vi "SearchArrayPath.vi"(6 "Current Direction (T=Positive)":bool=TRUE, 7 "Current Pos":T2, 8 "Target":T3, 9 "Blacklist":cluster{"X":dbl, "Y":dbl, "Z":dbl}[](array[cluster]), 10 "Path Taken":T1[](array[typedef]), 11 "All Lines":T4) -> (1 "Found Path?":bool, 2 "Path taken":T1[][](array[typedef]))   [LabVIEW 2014, in "Map Data.lvlib"]
uses:
  Map Data.lvlib
  All-Lines.ctl
  LineCluster.ctl
  LineConnection.ctl
  Components/PathFinder/Controls/PathControl.ctl
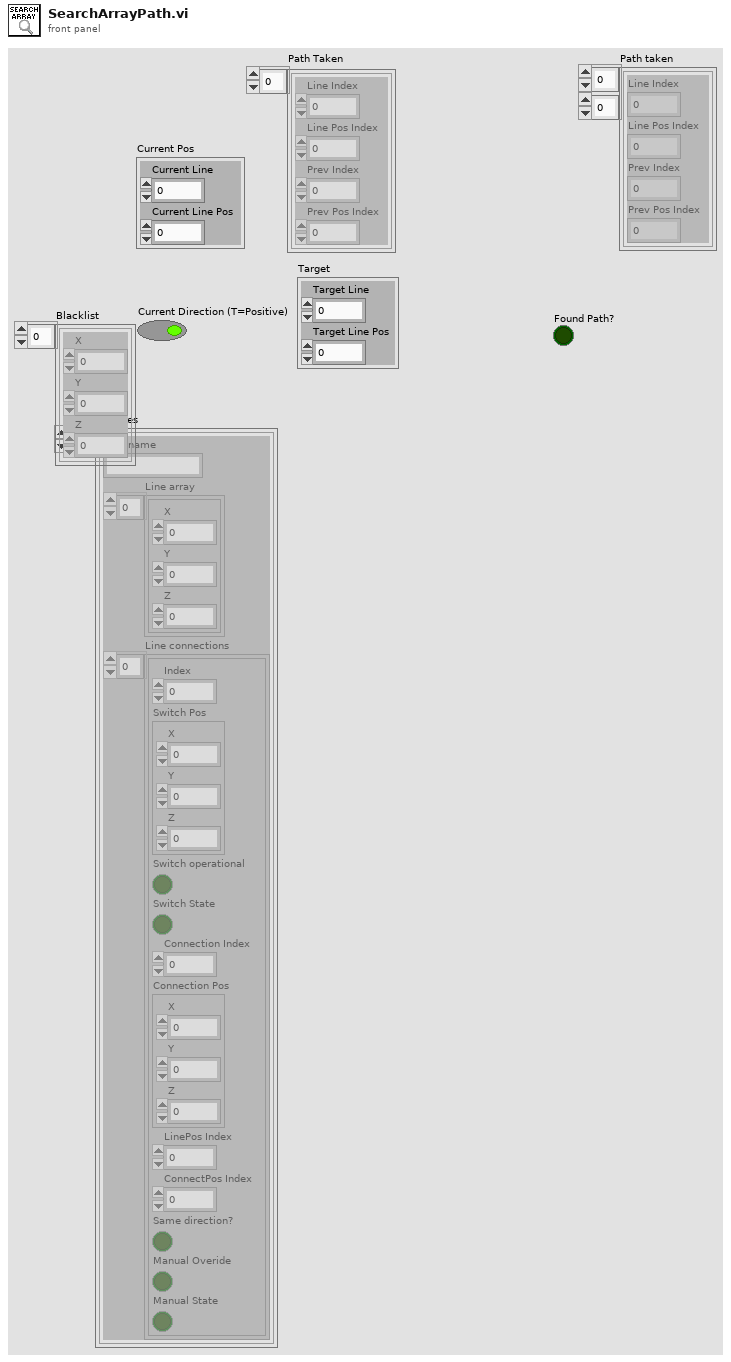
[diagram p1: front panel]
types:
  T1 = typedef "PathControl.ctl" = cluster{"Line Index":i32, "Line Pos Index ":i32, "Prev Index ":i32, "Prev Pos Index":i32}
  T2 = cluster{"Current Line":i32, "Current Line Pos":i32}
  T3 = cluster{"Target Line":i32, "Target Line Pos":i32}
  T4 = typedef "Map Data.lvlib/All-Lines.ctl" = T5[]
  T5 = typedef "Map Data.lvlib/LineCluster.ctl" = cluster{"Line name":string, "Line array":cluster{"X":dbl, "Y":dbl, "Z":dbl}[], "Line connections":T6[]}
  T6 = typedef "Map Data.lvlib/LineConnection.ctl" = cluster{"Index":i32, "Switch Pos":cluster{"X":dbl, "Y":dbl, "Z":dbl}, "Switch operational":bool, "Switch State":bool, "Connection Index":i32, "Connection Pos":cluster{"X":dbl, "Y":dbl, "Z":dbl}, "LinePos Index":i32, "ConnectPos Index":i32, "Same direction?":bool, "Manual Overide":bool, "Manual State":bool}
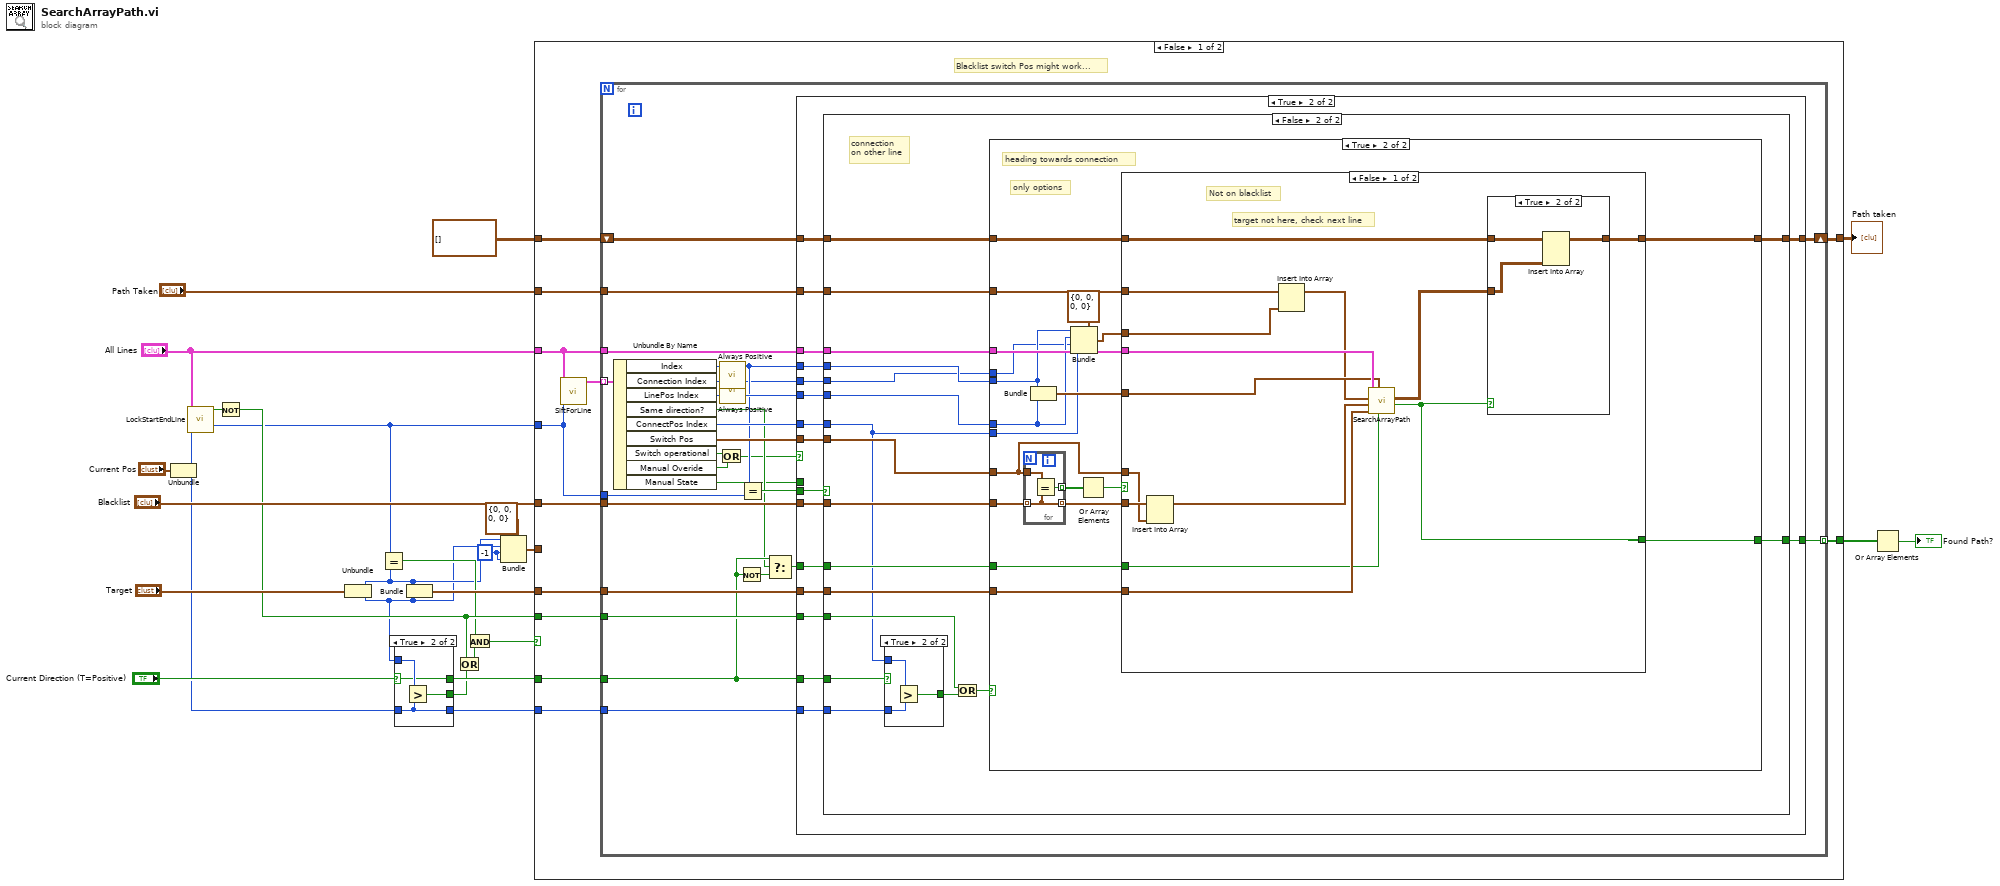
[diagram p0: block diagram]
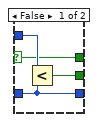
[diagram p2: hidden frame]
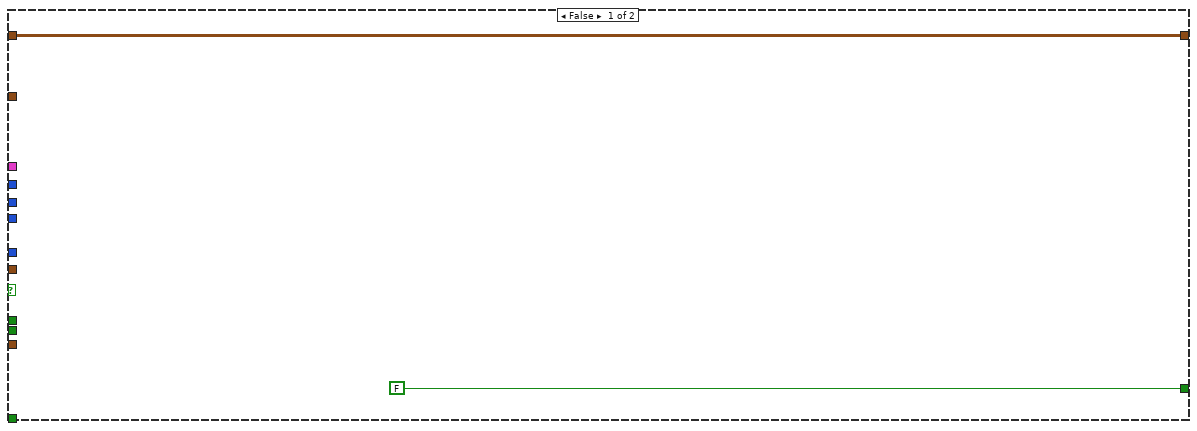
[diagram p3: hidden frame]
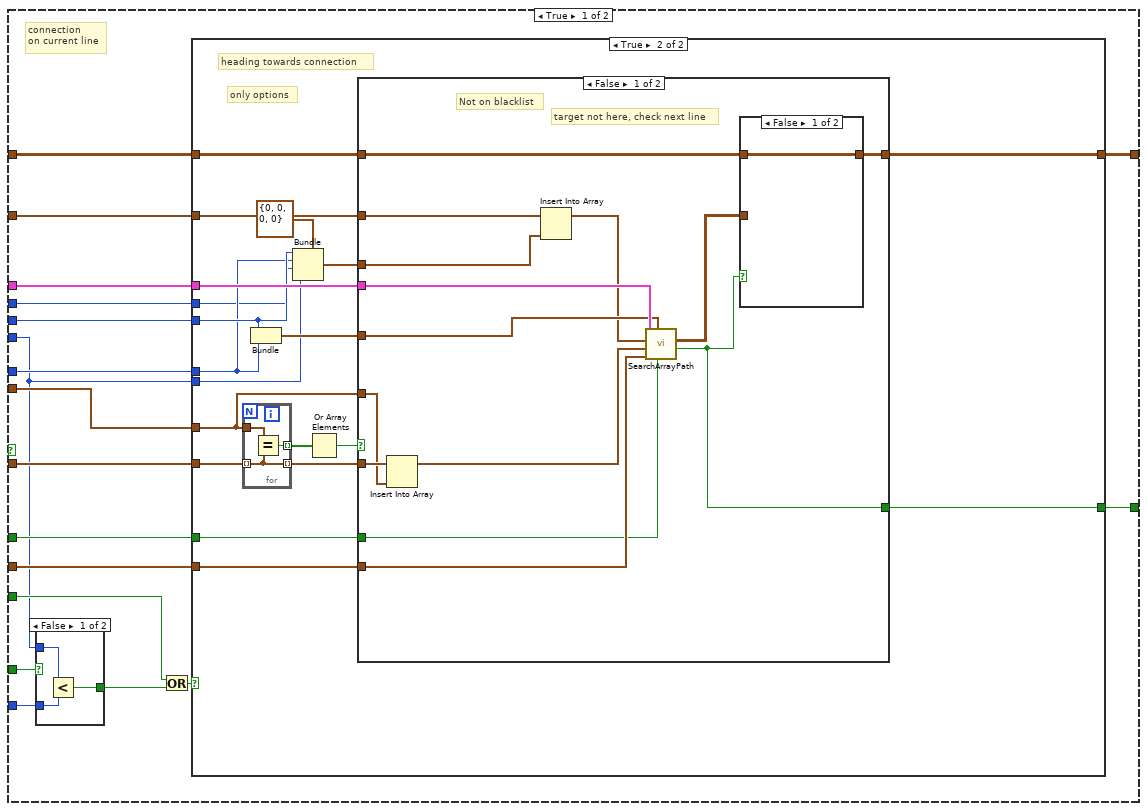
[diagram p4: hidden frame]
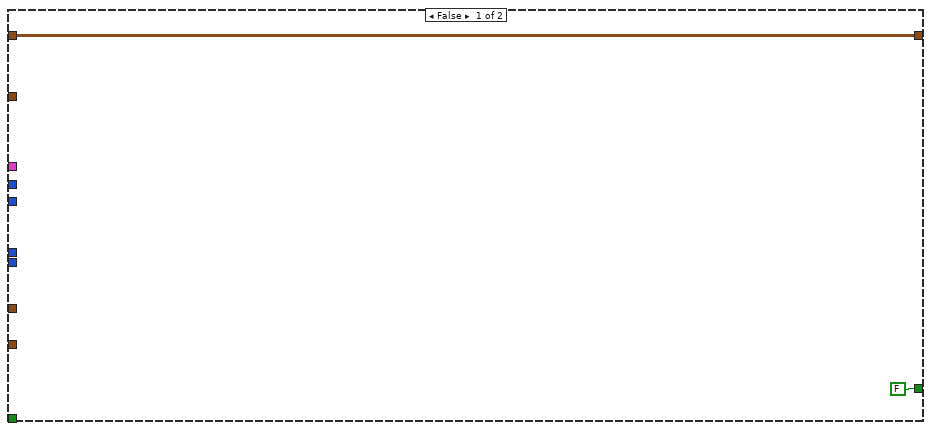
[diagram p5: hidden frame]
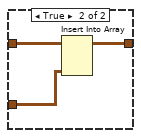
[diagram p6: hidden frame]
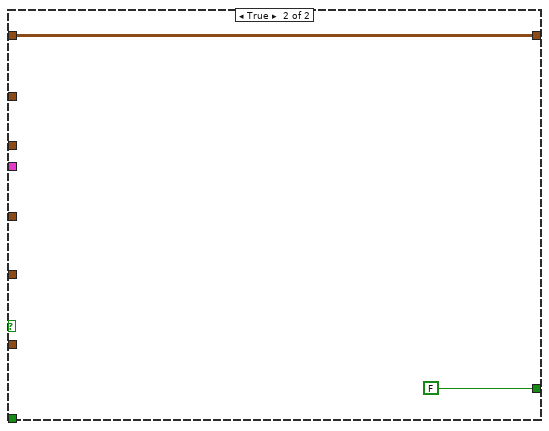
[diagram p7: hidden frame]
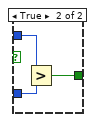
[diagram p8: hidden frame]
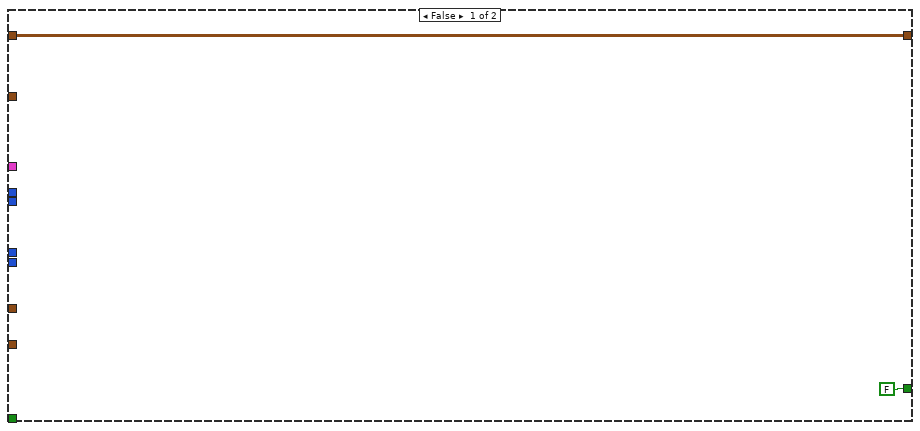
[diagram p9: hidden frame]
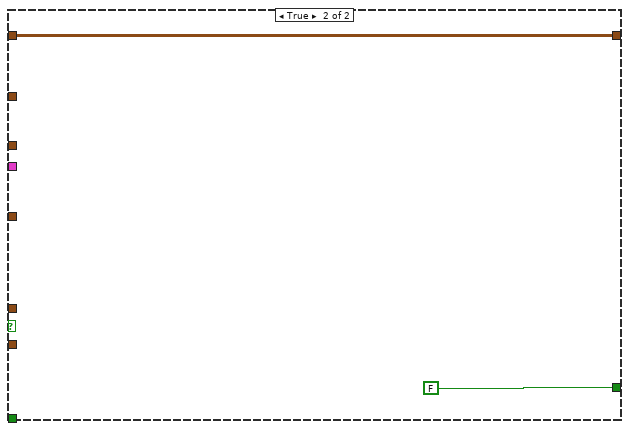
[diagram p11: hidden frame]
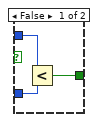
[diagram p12: hidden frame]
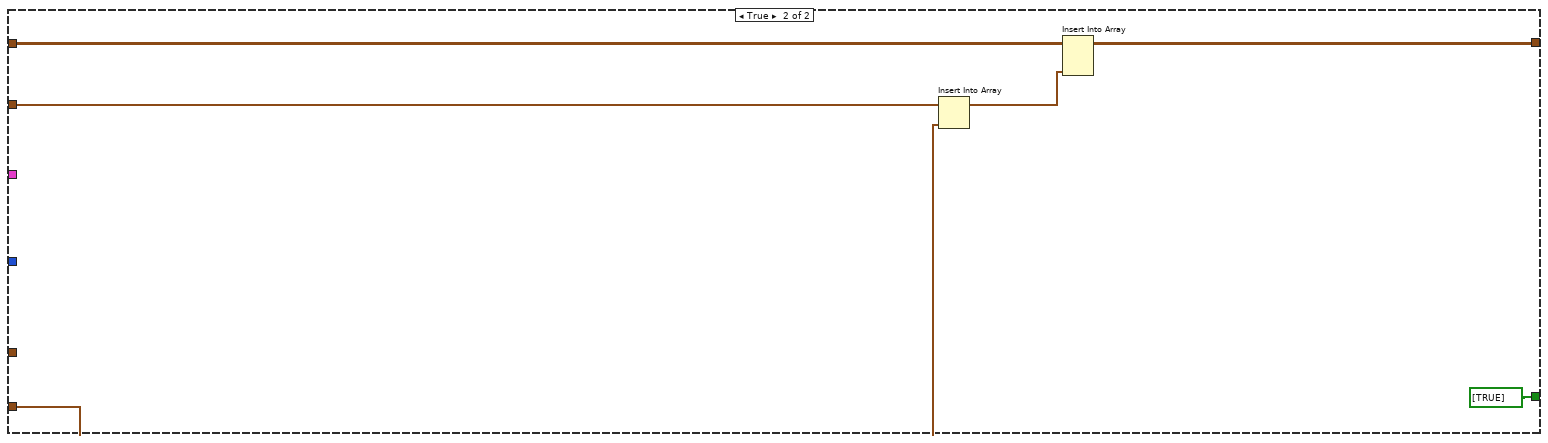
[diagram p13: hidden frame]
diagram:
  w3 = -1 ("Prev Pos Index")
  n1 = Unbundle("Current Pos") -> ("Current Line"=w12:i32, "Current Line Pos"=w17:i32)
  n2 = call "LockStartEndLine.vi"("index"=w12, "All Lines"="All Lines") -> ("Not Locked?"=w21:bool)  [unwired: 9 in]
  n3 = Not(x=w21) -> (.not. x?=w13:bool)
  n4 = Unbundle("Target") -> ("Target Line"=w5:i32, "Target Line Pos"=w4:i32)
  n5 = Equal?(x=w12, y=w5) -> (x = y?=w10:bool)
  n6 = case shown="True" "Current Direction (T=Positive)" {
    selector: "Current Direction (T=Positive)" -> [w28 w32]
    tunnel: w4 -> [w30 w34]
    tunnel: w17 -> [w27 w31]
    tunnel: [w29 w33] -> w14
    tunnel: [w28 w32] -> w15
    tunnel: [w27 w31] -> w16
    frame False {
      n7 = Less?(x=w30, y=w27) -> (x < y?=w29:bool)
    }
    frame True {
      n8 = Greater?(x=w34, y=w31) -> (0:w33:bool)
    }
  }
  n9 = Bundle("Target Line"=w5, "Target Line Pos"=w4) -> (w19:T3)  [unwired: 1 in]
  n10 = Or(x=w13, y=w14) -> (x .or. y?=w11:bool)
  n11 = And(x=w10, y=w11) -> (x .and. y?=w9:bool)
  n12 = Bundle(cluster=T1 {"Line Index"=0, "Line Pos Index "=0, "Prev Index "=0, "Prev Pos Index"=0} ("Posits 2"), "Line Index"=w5, "Line Pos Index"=w4, "Prev Index"=w3, "Prev Pos Index"=w3) -> (w2:T1)
  n13 = case shown="False" w9 {
    tunnel: "Path Taken" -> [w46 w234]
    tunnel: [w45 bool[] [TRUE]] -> w26
    tunnel: w15 -> [w44 _]
    tunnel: "Blacklist" -> [w43 _]
    tunnel: w16 -> [w42 _]
    tunnel: w13 -> [w41 _]
    tunnel: "All Lines" -> [w39 _]
    tunnel: w12 -> [w38 _]
    tunnel: w19 -> [w37 _]
    tunnel: T1[][] [] ("Path taken") -> [w36 w232]
    tunnel: [w35 w231] -> w1
    tunnel: w2 -> [_ w229]
    frame False {
      # "Blacklist switch Pos might work..."
      n14 = call "SiftForLine.vi"("Current Line"=w38, "All Lines"=w39) -> ("Line connections"=w40:T6[])  [unwired: 9 in]
      n15 = for {
        tunnel: w40 -> [w71] mode=indexing
        tunnel: w43 -> [w72]
        tunnel: [w69] -> w45 mode=indexing
        tunnel: w39 -> [w70]
        tunnel: w46 -> [w73]
        tunnel: w44 -> [w55]
        tunnel: w42 -> [w68]
        tunnel: w41 -> [w64]
        tunnel: w38 -> [w63]
        tunnel: w37 -> [w57]
        shift-right: [w52] -> w35
        shift-left: w36 -> [w51]
        n16 = Unbundle By Name(w71) -> ("Index"=w62:i32, "Connection Index"=w60:i32, "LinePos Index"=w67:i32, "Same direction?"=w53:bool, "ConnectPos Index"=w65:i32, "Switch Pos"=w66:cluster{"X":dbl, "Y":dbl, "Z":dbl}, "Switch operational"=w50:bool, "Manual Overide"=w49:bool, "Manual State"=w47:bool)
        n17 = Or(x=w50, y=w49) -> (x .or. y?=w48:bool)
        n18 = call "Always Positive.vi"("Input"=w62) -> ("Output"=w61:i32)  [unwired: 8 in]
        n19 = call "Always Positive.vi"("Input"=w60) -> ("Output"=w59:i32)  [unwired: 8 in]
        n20 = Not(x=w55) -> (.not. x?=w56:bool)
        n21 = Equal?(x=w61, y=w63) -> (x = y?=w58:bool)
        n22 = Select(t=w55, s=w53, f=w56) -> (s? t:f=w54:bool)
        n23 = case shown="True" w48 {
          tunnel: w73 -> [_ w92]
          tunnel: w72 -> [_ w91]
          tunnel: w70 -> [_ w90]
          tunnel: [FALSE ("Found Path?") w89] -> w69
          tunnel: w68 -> [_ w88]
          tunnel: w67 -> [_ w87]
          tunnel: w66 -> [_ w86]
          tunnel: w65 -> [_ w85]
          tunnel: w64 -> [_ w84]
          tunnel: w61 -> [_ w83]
          tunnel: w59 -> [_ w82]
          tunnel: w58 -> [_ w81]
          tunnel: w57 -> [_ w80]
          tunnel: w55 -> [_ w79]
          tunnel: w54 -> [_ w78]
          tunnel: [w74 w77] -> w52
          tunnel: w51 -> [w74 w76]
          tunnel: w47 -> [_ _]
          frame False {
          }
          frame True {
            n24 = case shown="False" w81 {
              tunnel: w92 -> [w110 w178]
              tunnel: w82 -> [w109 w162]
              tunnel: w91 -> [w108 w177]
              tunnel: w90 -> [w107 w176]
              tunnel: [w106 w175] -> w89
              tunnel: w79 -> [w105 w174]
              tunnel: w88 -> [w104 w173]
              tunnel: w87 -> [w93 w167]
              tunnel: w86 -> [w103 w172]
              tunnel: w85 -> [w102 w161]
              tunnel: w84 -> [w99 w169]
              tunnel: w83 -> [w94 w168]
              tunnel: w80 -> [w98 w166]
              tunnel: w78 -> [w97 w165]
              tunnel: [w96 w163] -> w77
              tunnel: w76 -> [w95 w164]
              frame True {
                # "connection \non current line"
                n25 = case shown="False" w105 {
                  tunnel: w93 -> [w156 w159]
                  tunnel: w104 -> [w155 w158]
                  tunnel: [w157 w160] -> w100
                  frame False {
                    n26 = Less?(x=w156, y=w155) -> (x < y?=w157:bool)
                  }
                  frame True {
                    n27 = Greater?(x=w159, y=w158) -> (0:w160:bool)
                  }
                }
                n28 = Or(x=w99, y=w100) -> (x .or. y?=w101:bool)
                n29 = case shown="True" w101 {
                  tunnel: w110 -> [_ w131]
                  tunnel: w109 -> [_ w116]
                  tunnel: w108 -> [_ w129]
                  tunnel: w107 -> [_ w128]
                  tunnel: [FALSE ("Found Path?") w127] -> w106
                  tunnel: w103 -> [_ w123]
                  tunnel: w102 -> [_ w115]
                  tunnel: w98 -> [_ w122]
                  tunnel: w97 -> [_ w121]
                  tunnel: [w111 w120] -> w96
                  tunnel: w95 -> [w111 w119]
                  tunnel: w94 -> [_ w114]
                  tunnel: w93 -> [_ w113]
                  frame False {
                  }
                  frame True {
                    # "only options"
                    # "heading towards connection"
                    n30 = for {
                      tunnel: w129 -> [w134] mode=indexing
                      tunnel: w123 -> [w132]
                      tunnel: [w133] -> w126 mode=indexing
                      tunnel: [w134] -> w125 mode=indexing
                      n31 = Equal?(x=w132, y=w134) -> (x = y?=w133:bool)
                    }
                    n32 = Bundle("Output"=w116, "ConnectPos Index"=w115) -> (w124:cluster{"Output":i32, "ConnectPos Index":i32})  [unwired: 1 in]
                    n33 = Bundle(cluster=T1 {"Line Index"=0, "Line Pos Index "=0, "Prev Index "=0, "Prev Pos Index"=0} ("Posits 2"), "Line Index"=w116, "Line Pos Index"=w115, "Prev Index"=w114, "Prev Pos Index"=w113) -> (w117:T1)
                    n34 = Or Array Elements(Boolean array=w126) -> (logical OR=w130:bool)
                    n35 = case shown="False" w130 {
                      tunnel: w131 -> [w148 _]
                      tunnel: w125 -> [w145 _]
                      tunnel: w122 -> [w147 _]
                      tunnel: [w136 FALSE] -> w127
                      tunnel: w128 -> [w146 _]
                      tunnel: w123 -> [w143 _]
                      tunnel: w124 -> [w142 _]
                      tunnel: w121 -> [w140 _]
                      tunnel: [w137 w153] -> w120
                      tunnel: w119 -> [w138 w153]
                      tunnel: w117 -> [w135 _]
                      frame False {
                        # "target not here, check next line"
                        # "Not on blacklist"
                        n36 = Insert Into Array(array=w145, new element=w143) -> (w144:cluster{"X":dbl, "Y":dbl, "Z":dbl}[])  [unwired: 1 in]
                        n37 = Insert Into Array(array=w148, new element=w135) -> (w141:T1[])  [unwired: 1 in]
                        n38 = call "SearchArrayPath.vi"("Current Direction (T=Positive)"=w140, "Current Pos"=w142, "Target"=w147, "Blacklist"=w144, "Path Taken"=w141, "All Lines"=w146) -> ("Found Path?"=w136:bool, "Path taken"=w139:T1[][])  [unwired: 4 in]
                        n39 = case shown="False" w136 {
                          tunnel: w139 -> [_ w150]
                          tunnel: w138 -> [w149 w151]
                          tunnel: [w149 w152] -> w137
                          frame False {
                          }
                          frame True {
                            n40 = Insert Into Array(array=w151, new element=w150) -> (w152:T1[][])  [unwired: 2 in]
                          }
                        }
                      }
                      frame True {
                      }
                    }
                  }
                }
              }
              frame False {
                # "connection\non other line"
                n41 = case shown="True" w174 {
                  tunnel: w161 -> [w224 w227]
                  tunnel: w173 -> [w223 w226]
                  tunnel: [w225 w228] -> w170
                  frame False {
                    n42 = Less?(x=w224, y=w223) -> (x < y?=w225:bool)
                  }
                  frame True {
                    n43 = Greater?(x=w227, y=w226) -> (0:w228:bool)
                  }
                }
                n44 = Or(x=w169, y=w170) -> (x .or. y?=w171:bool)
                n45 = case shown="True" w171 {
                  tunnel: w178 -> [_ w186]
                  tunnel: w168 -> [_ w184]
                  tunnel: w177 -> [_ w198]
                  tunnel: w176 -> [_ w197]
                  tunnel: [FALSE ("Found Path?") w196] -> w175
                  tunnel: w172 -> [_ w192]
                  tunnel: w167 -> [_ w183]
                  tunnel: w166 -> [_ w191]
                  tunnel: w165 -> [_ w190]
                  tunnel: w164 -> [w179 w189]
                  tunnel: [w179 w188] -> w163
                  tunnel: w162 -> [_ w182]
                  tunnel: w161 -> [_ w181]
                  frame False {
                  }
                  frame True {
                    # "only options"
                    # "heading towards connection"
                    n46 = for {
                      tunnel: w198 -> [w202] mode=indexing
                      tunnel: w192 -> [w200]
                      tunnel: [w201] -> w195 mode=indexing
                      tunnel: [w202] -> w194 mode=indexing
                      n47 = Equal?(x=w200, y=w202) -> (x = y?=w201:bool)
                    }
                    n48 = Bundle("Output"=w184, "LinePos Index"=w183) -> (w193:cluster{"Output":i32, "LinePos Index":i32})  [unwired: 1 in]
                    n49 = Bundle(cluster=T1 {"Line Index"=0, "Line Pos Index "=0, "Prev Index "=0, "Prev Pos Index"=0} ("Posits 2"), "Line Index"=w184, "Line Pos Index"=w183, "Prev Index"=w182, "Prev Pos Index"=w181) -> (w187:T1)
                    n50 = Or Array Elements(Boolean array=w195) -> (logical OR=w199:bool)
                    n51 = case shown="False" w199 {
                      tunnel: w186 -> [w216 _]
                      tunnel: w194 -> [w213 _]
                      tunnel: w191 -> [w215 _]
                      tunnel: [w207 FALSE] -> w196
                      tunnel: w197 -> [w214 _]
                      tunnel: w192 -> [w211 _]
                      tunnel: w193 -> [w210 _]
                      tunnel: w190 -> [w208 _]
                      tunnel: w189 -> [w206 w221]
                      tunnel: [w205 w221] -> w188
                      tunnel: w187 -> [w203 _]
                      frame False {
                        # "target not here, check next line"
                        # "Not on blacklist"
                        n52 = Insert Into Array(array=w213, new element=w211) -> (w212:cluster{"X":dbl, "Y":dbl, "Z":dbl}[])  [unwired: 1 in]
                        n53 = Insert Into Array(array=w216, new element=w203) -> (w209:T1[])  [unwired: 1 in]
                        n54 = call "SearchArrayPath.vi"("Current Direction (T=Positive)"=w208, "Current Pos"=w210, "Target"=w215, "Blacklist"=w212, "Path Taken"=w209, "All Lines"=w214) -> ("Found Path?"=w207:bool, "Path taken"=w204:T1[][])  [unwired: 4 in]
                        n55 = case shown="True" w207 {
                          tunnel: w206 -> [w217 w219]
                          tunnel: [w217 w220] -> w205
                          tunnel: w204 -> [_ w218]
                          frame False {
                          }
                          frame True {
                            n56 = Insert Into Array(array=w219, new element=w218) -> (w220:T1[][])  [unwired: 2 in]
                          }
                        }
                      }
                      frame True {
                      }
                    }
                  }
                }
              }
            }
          }
        }
      }
    }
    frame True {
      n57 = Insert Into Array(array=w234, new element=w229) -> (w230:T1[])  [unwired: 1 in]
      n58 = Insert Into Array(array=w232, new element=w230) -> (w231:T1[][])  [unwired: 2 in]
    }
  }
  "Path taken" <- w1
  n59 = Or Array Elements(Boolean array=w26) -> (logical OR=→"Found Path?":bool)
